vi "Memory.Pointer.I64.Write.0D.vi"(8 "error in (no error)":errorcluster, 9 "offset (0)":u64 format="%d bytes", 10 "value in":i64, 11 "pointer in":refnum<class "Memory.Pointer.I64.lvclass">) -> (0 "error out":errorcluster, 1 "offset out":u64 format="%d bytes", 2 "value out":i64, 3 "pointer out":refnum<class "Memory.Pointer.I64.lvclass">)   [LabVIEW 2016, in "Memory.lvlib" / "Memory.Pointer.I64.lvclass"]
uses:
  Memory.Pointer.I64.lvclass
  C:/Git/SourceTree/DSF/Source/Submodules/Memory/Source/Classes/Pointer/Memory.Pointer.lvclass
  Pointer/Memory.Pointer.lvclass/Memory.Pointer.ctl
  Pointer/Memory.Pointer.Write.Safe.0D.I64.vi
  Pointer/Memory.Pointer.Write.Unsafe.0D.I64.vi
  Pointer/Memory.Pointer.Parameter Check.Null Pointer.vi
  Pointer/Memory.Pointer.Parameter Check.Subset.vi
  Pointer/Memory.Pointer.Get Address.vi
  Pointer/Memory.Pointer.Errors.vi
  Pointer/Memory.Pointer.Errors.Null Pointer.vi
  Pointer/Memory.Pointer.Errors.Out of Bounds.vi
  Pointer/Memory.Pointer.Get Size.vi
  Pointer/Memory.Pointer.Errors.Create Error.vi
  Submodules/SEH/Source/VIs/Static Error Handling.Source Buffer.Write.String.vi
  Pointer/Memory.Pointer.Errors.Write Pointer Size.vi
  Submodules/SEH/Source/VIs/Static Error Handling.Source Buffer.Write.Numeric.Scalar.Base10.vi
  Submodules/SEH/Source/VIs/Static Error Handling.Source Buffer.Write.Numeric.Scalar.Base10 (U64).vi
  Submodules/SEH/Source/VIs/Static Error Handling.Error Cluster Constant.vi
  Submodules/SEH/Source/VIs/Static Error Handling.Error Cluster Constant (256B).vi
  Submodules/SEH/Source/VIs/Static Error Handling.Parameters.Status.Set.vi
  Submodules/SEH/Source/VIs/Static Error Handling.Parameters.Code.Set.vi
  Submodules/SEH/Source/VIs/Static Error Handling.Parameters.VI Source.Set.vi
  Constants/Memory.Constants.vi
  Constants/Memory.Constants.Library Name.vi
  Pointer/Memory.Pointer.Errors.Get Info.vi
  Pointer/Memory.Pointer.lvclass
  C:/Git/SourceTree/DSF/Source/Submodules/Memory/Source/Classes/Internal/Memory.Pointer.Internal.lvclass
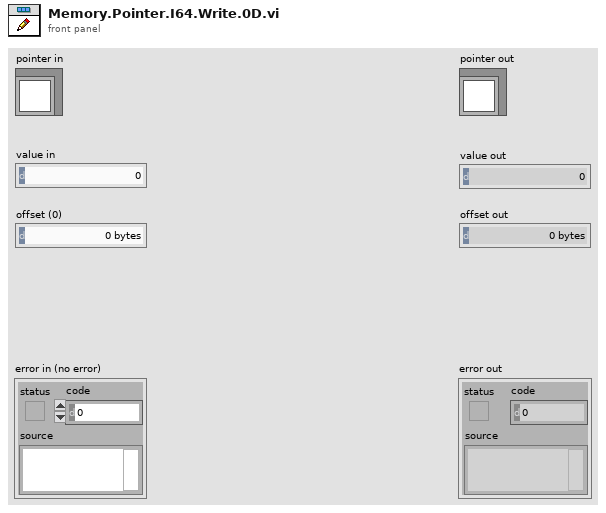
[diagram p1: front panel]
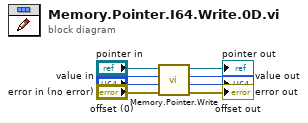
[diagram p0: block diagram]
diagram:
  n1 = call-poly "Memory.Pointer.Write.vi"("error in (no error)"="error in (no error)", "offset (0)"="offset (0)", "value"="value in", "pointer in"="pointer in") -> ("error out"=→"error out":errorcluster, "offset out"=→"offset out":u64, "value"=→"value out":i64, "pointer out"=→"pointer out":refnum<class "Memory.Pointer.I64.lvclass">)  [unwired: 4 in]
